vi "ObjRef to NodeRef.vi"(3 "ObjectRef":refnum<data-value>) -> (1 "NodeRef":refnum<data-value>)   [LabVIEW 2020, in "PicoG-ParserLexer.lvlib" / "Node.lvclass"]
uses:
  Node.lvclass
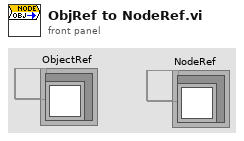
[diagram p1: front panel]
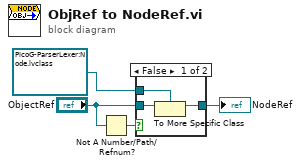
[diagram p0: block diagram]
diagram:
  n1 = Not A Number/Path/Refnum?(number/path/refnum="ObjectRef") -> (NaN/Path/Refnum?=w4:bool)
  n2 = case shown="False" w4 {
    tunnel: "ObjectRef" -> [w7 _]
    tunnel: refnum<data-value> refnum ("NodeRef") -> [w6 _]
    tunnel: [w5 _] -> w1
    frame False {
      n3 = To More Specific Class(target class=w6, reference=w7) -> (specific class reference=w5:refnum<data-value>)  [unwired: 1 in, 1 out]
    }
    frame True {
    }
  }
  "NodeRef" <- w1
